vi "Shapelet Transform.vi"() -> ()   [LabVIEW 2016]
uses:
  _Shapelets Search (Brute Force)/Shapelets Search (Brute Force).lvlib
panel:
  in  "Number of Shapelets":i32 caption="Число шейплетов"
  in  "Number of Channels":i32 caption="Число каналов"
  in  "Exit":bool
  in  "Save Data":bool
  out "Number of Trials":i32 caption="Число проб в файле"
  out "Progress":i32(slide) caption="Процесс преобразования" min=0 max=288 scale=0.0..222.0
  in  "Shapelets File Path":path caption="Путь к файлу с набором шейплетов"
  in  "Data File Path":path caption="Путь к файлу с данными"
  # "This VI is a part of BCI Design library, http://www.ru-bci.org \nCopyright © 2020, Sotnikov Peter, All rights reserved. License: GNU GPLv3"
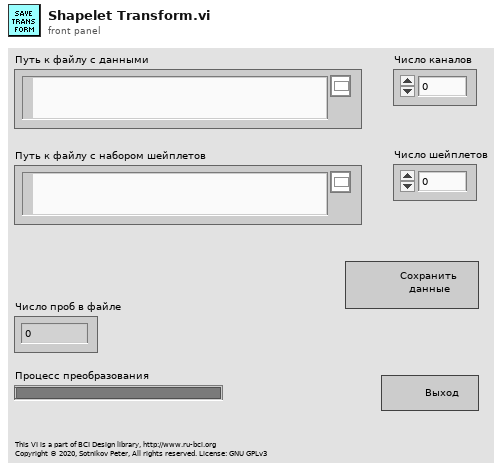
[diagram p1: front panel]
types:
  T1 = cluster{"Number of Trials":refnum<vi>, "Progress":refnum<vi>}
  T2 = cluster{"ClassLabel":string, "FeatureVector":dbl[][]}[]
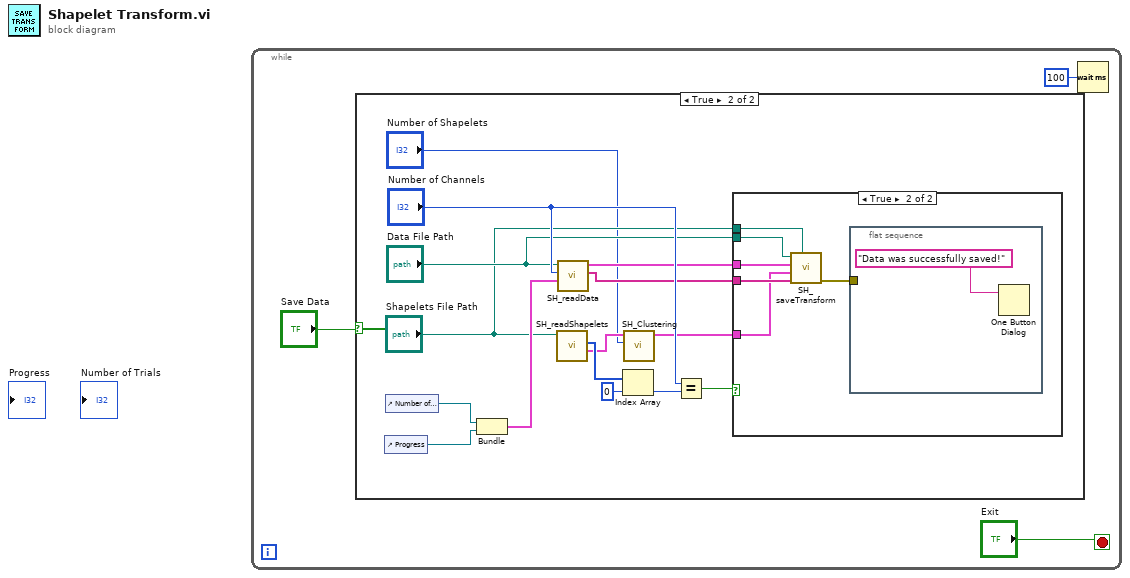
[diagram p0: block diagram]
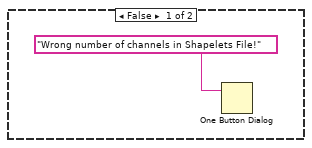
[diagram p3: hidden frame]
diagram:
  n1 = while {
    stop <- "Exit" stop-if-true
    n2 = case shown="True" "Save Data" {
      frame False {
      }
      frame True {
        n3 = control-ref of="Progress"() -> (w17:refnum<vi>)
        n4 = control-ref of="Number of Trials"() -> (w18:refnum<vi>)
        n5 = Bundle("Number of Trials"=w18, "Progress"=w17) -> (w16:T1)  [unwired: 1 in]
        n6 = call "SH_readShapelets.vi"("Shapelets File"="Shapelets File Path") -> ("Array of Shapelets"=w6:cluster{dbl[][]}[], "size(s)"=w15:i32[])  [unwired: 8 in, 1 out]
        n7 = call "SH_readData.vi"("ControlRefs"=w16, "NumberOfChannels"="Number of Channels", "Data File"="Data File Path") -> ("CLassLabels out"=w9:string[], "ArrayOfTrials"=w10:T2)  [unwired: 6 in, 1 out]
        n8 = Index Array(array=w15, index=0) -> (element=w13:i32)
        n9 = call "SH_Clustering.vi"("Array of Shapelets in"=w6, "NumberOfShapelets"="Number of Shapelets") -> ("Array of Shapelets out"=w5:cluster{dbl[][]}[])  [unwired: 6 in, 2 out]
        n10 = Equal?(x="Number of Channels", y=w13) -> (x = y?=w11:bool)
        n11 = case shown="True" w11 {
          tunnel: "Data File Path" -> [_ w25]
          tunnel: w10 -> [_ w24]
          tunnel: w5 -> [_ w20]
          tunnel: w9 -> [_ w23]
          tunnel: "Shapelets File Path" -> [_ w21]
          frame False {
            n12 = One Button Dialog(message="Wrong number of channels in Shapelets File!") -> ()  [unwired: 1 in, 1 out]
          }
          frame True {
            n13 = call "SH_saveTransform.vi"("Shapelets File"=w21, "CLassLabels out"=w23, "Array of Shapelets"=w20, "ArrayOfTrials"=w24, "Data File"=w25) -> ("error out"=w22:errorcluster)  [unwired: 6 in]
            n14 = flat-sequence {
              tunnel: w22 -> [_]
              frame #0 {
                n15 = One Button Dialog(message="Data was successfully saved!") -> ()  [unwired: 1 in, 1 out]
              }
            }
          }
        }
      }
    }
    n16 = Wait (ms)(milliseconds to wait=u32 100) -> ()  [unwired: 1 out]
  }
